vi "Write Data Entry Limits Minimum.vi"(8 "error in (no error)":errorcluster, 10 "Minimum":dbl, 11 "Numeric.lvclass in":refnum<class "Numeric.lvclass">) -> (0 "error out":errorcluster, 3 "Numeric.lvclass out":refnum<class "Numeric.lvclass">)   [LabVIEW 2015, in "Numeric.lvclass"]
uses:
  Numeric.lvclass
  Numeric.lvclass/Numeric.ctl
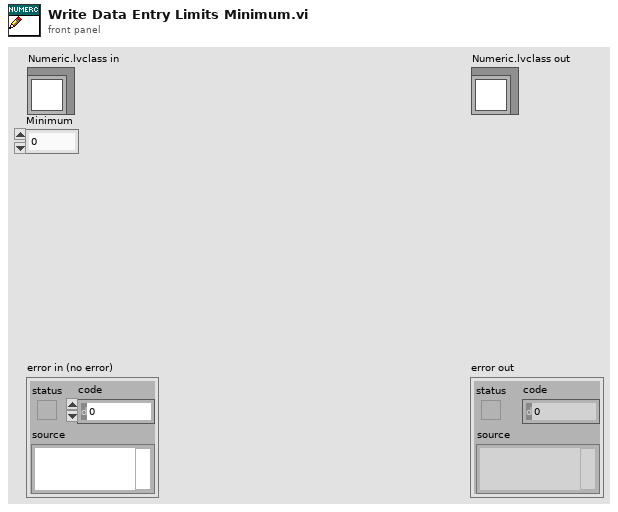
[diagram p1: front panel]
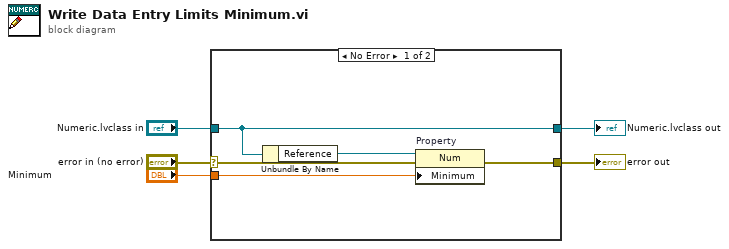
[diagram p0: block diagram]
diagram:
  n1 = case shown="No Error" "error in (no error)" {
    selector: "error in (no error)" -> [w6 w12]
    tunnel: [w10 w12] -> w4
    tunnel: [w8 w11] -> w2
    tunnel: "Numeric.lvclass in" -> [w8 w11]
    tunnel: "Minimum" -> [w9 _]
    frame No Error {
      n2 = Unbundle By Name(w8) -> ("Reference"=w7:refnum<vi>)
      n3 = property on="Property" class="Num"(reference=w7, error in=w6, "Minimum"=w9) -> (error out=w10:errorcluster)  [unwired: 1 out]
    }
    frame Error {
    }
  }
  "error out" <- w4
  "Numeric.lvclass out" <- w2
